vi "Get Path Regex.vi"(8 "error in (no error)":errorcluster, 11 "Challenges in":refnum<class "Challenges.lvclass">) -> (0 "error out":errorcluster, 2 "Path Regex":string, 3 "Challenges out":refnum<class "Challenges.lvclass">)   [LabVIEW 2020, in "Summer of LabVIEW.lvlib" / "Challenges.lvclass"]
uses:
  Challenges.lvclass
  Challenges.lvclass/Challenges.ctl
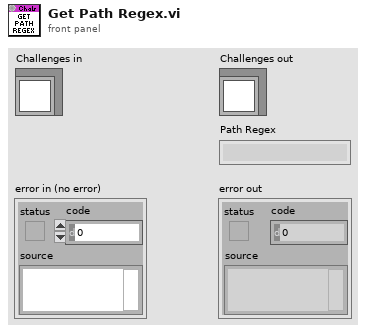
[diagram p1: front panel]
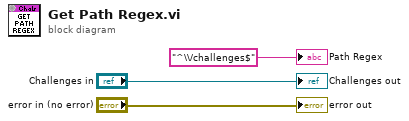
[diagram p0: block diagram]
diagram:
  "error out" <- "error in (no error)"
  "Challenges out" <- "Challenges in"
  "Path Regex" <- "^\\/challenges$" ("Path Regex")
